vi "DataManagementUpdateTrendAnnotationIdRoutedMessage_Name.vi"() -> (1 "MessageName":string)   [LabVIEW 2017]
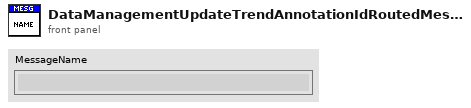
[diagram p1: front panel]
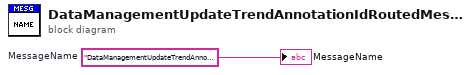
[diagram p0: block diagram]
diagram:
  w1 = "DataManagementUpdateTrendAnnotationIdRoutedMessage"  # MessageName
  "MessageName" <- w1
